vi "create calibration file name.vi"(11 "Folder Calibraion":string[](array[string])) -> (3 "Name file":string[](array[string]))   [LabVIEW 2015]
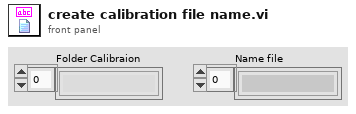
[diagram p1: front panel]
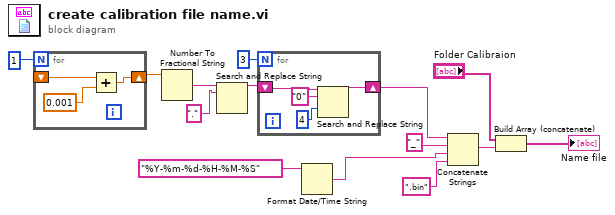
[diagram p0: block diagram]
diagram:
  n1 = for {
    N: 1 -> [_]
    shift-right: [w15] -> w11
    shift-left: _ -> [w16]
    n2 = Add(x=w16, y=0.001) -> (x+y=w15:dbl)
  }
  n3 = Number To Fractional String(number=w11) -> (F-format string=w7:string)  [unwired: 3 out]
  n4 = Search and Replace String(input string=w7, search string="." ("replace string (\"\")")) -> (result string=w9:string)  [unwired: 1 in, 8 out]
  n5 = for {
    N: 3 -> [_]
    shift-right: [w20] -> w6
    shift-left: w9 -> [w18]
    n6 = Search and Replace String(input string=w18, search string="0", offset=4 ("offset (0)")) -> (result string=w20:string)  [unwired: 1 in, 7 out]
  }
  n7 = Format Date/Time String(time format string (%c)="%Y-%m-%d-%H-%M-%S") -> (date/time string=w5:string)  [unwired: 2 in]
  n8 = Concatenate Strings(w6, "_" ("replace string (\"\")"), w5, ".bin" ("string")) -> (w13:string)
  n9 = Build Array (concatenate)("Folder Calibraion", w13) -> (→"Name file":string[])
